vi "ASI_change_Z_backlash.vi"(2 "error in (no error)":errorcluster, 3 "VISA resource name":refnum<visa-resource-name>="COM7", 4 "backlash (um)":dbl) -> (0 "error out":errorcluster, 1 "VISA resource name out":refnum<visa-resource-name>)   [LabVIEW 2015]
uses:
  <vilib>/Instr/_visa.llb/VISA Flush IO Buffer Mask.ctl
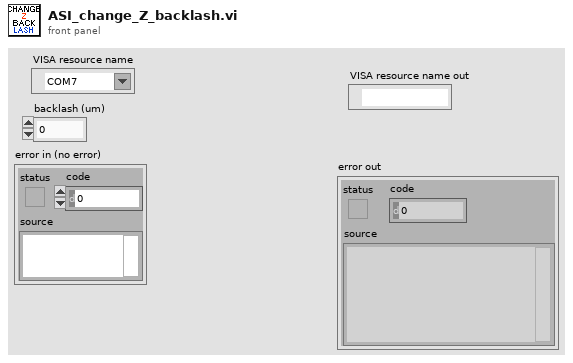
[diagram p1: front panel]
types:
  T1 = typedef "VISA Flush IO Buffer Mask.ctl" = u16
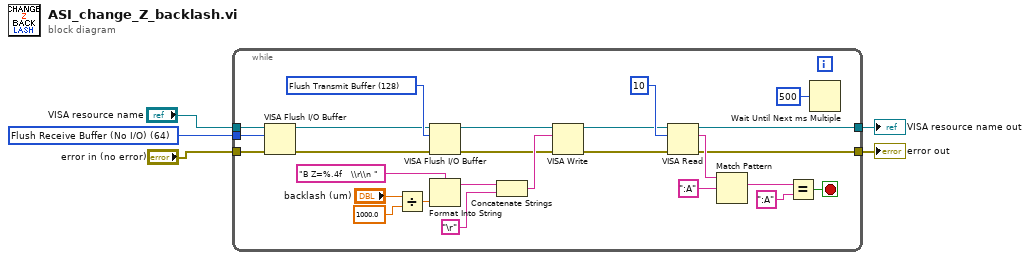
[diagram p0: block diagram]
diagram:
  w4 = T1 64 items=["Flush Receive Buffer"=16, "Write Transmit Buffer to Device"=32, "Flush Receive Buffer (No I/O)"=64, "Flush Transmit Buffer"=128] ("Mask")
  n1 = while {
    tunnel: "error in (no error)" -> [w28]
    tunnel: w4 -> [w22]
    tunnel: "VISA resource name" -> [w21]
    tunnel: [w13] -> w2
    tunnel: [w6] -> w1
    stop <- w12 stop-if-true
    w25 = T1 128 items=["Flush Receive Buffer"=16, "Write Transmit Buffer to Device"=32, "Flush Receive Buffer (No I/O)"=64, "Flush Transmit Buffer"=128] ("Mask")
    n2 = VISA Flush I/O Buffer(VISA resource name=w21, mask (16)=w22, error in (no error)=w28) -> (VISA resource name out=w24:refnum<visa-resource-name>, error out=w23:errorcluster)
    n3 = Divide(x="backlash (um)", y=1000.0) -> (x/y=w9:dbl)
    n4 = VISA Flush I/O Buffer(VISA resource name=w24, mask (16)=w25, error in (no error)=w23) -> (VISA resource name out=w27:refnum<visa-resource-name>, error out=w26:errorcluster)
    n5 = Format Into String(format string="B Z=%.4f   \\r\\n ", w9) -> (resulting string=w29:string)  [unwired: 2 in, 1 out]
    n6 = Concatenate Strings(w29, "\r") -> (w30:string)
    n7 = VISA Write(VISA resource name=w27, write buffer=w30, error in (no error)=w26) -> (VISA resource name out=w10:refnum<visa-resource-name>, error out=w14:errorcluster)  [unwired: 1 out]
    n8 = VISA Read(VISA resource name=w10, byte count=u32 10, error in (no error)=w14) -> (VISA resource name out=w6:refnum<visa-resource-name>, read buffer=w17:string, error out=w13:errorcluster)  [unwired: 1 out]
    n9 = Match Pattern(string=w17, regular expression=":A" ("y")) -> (match substring=w18:string)  [unwired: 1 in, 3 out]
    n10 = Equal?(x=w18, y=":A") -> (x = y?=w12:bool)
    n11 = Wait Until Next ms Multiple(millisecond multiple=u32 500) -> ()  [unwired: 1 out]
  }
  "error out" <- w2
  "VISA resource name out" <- w1
